vi "Main Engine Response LV2GBL.vi"(6 "Options":T1, 8 "error in":errorcluster) -> (0 "error out":errorcluster, 2 "Response":i32, 3 "Update":i32)   [LabVIEW 2021]
uses:
  Controls/Main Engine Engine No.Options.ctl
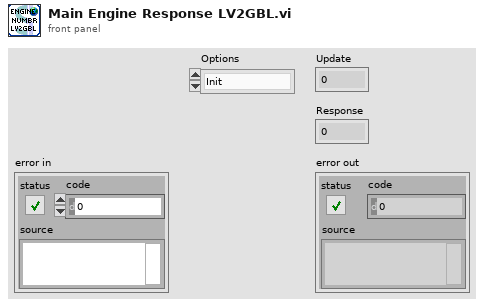
[diagram p1: front panel]
types:
  T1 = typedef "Main Engine Engine No.Options.ctl" = enum16{"Init", "Update", "Response", "Get"}
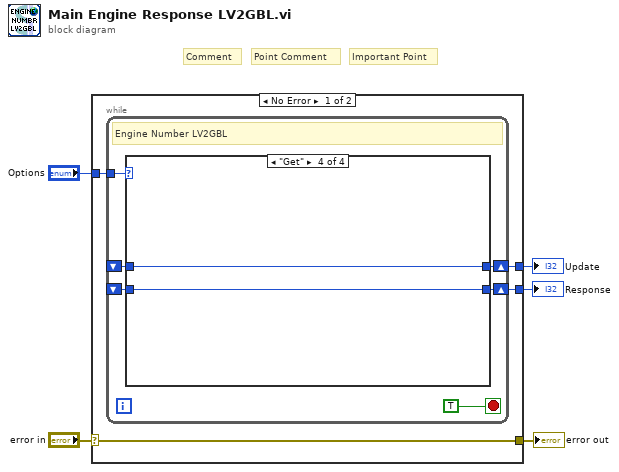
[diagram p0: block diagram]
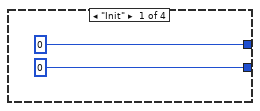
[diagram p2: hidden frame]
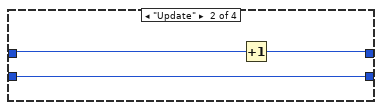
[diagram p3: hidden frame]
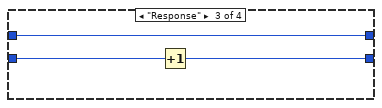
[diagram p4: hidden frame]
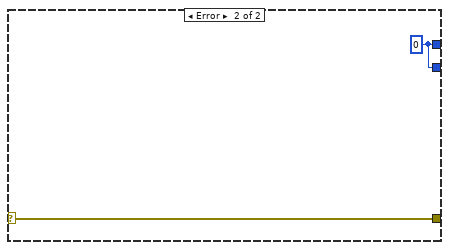
[diagram p5: hidden frame]
diagram:
  # "Important Point"
  # "Point Comment"
  # "Comment"
  n1 = case shown="No Error" "error in" {
    selector: "error in" -> [w8 w27]
    tunnel: "Options" -> [w9 _]
    tunnel: [w8 w27] -> w3
    tunnel: [w7 w26] -> w2
    tunnel: [w6 w26] -> w1
    frame No Error {
      n2 = while {
        tunnel: w9 -> [w14]
        shift-right: [w12] -> w6
        shift-left: _ -> [w10]
        shift-right: [w13] -> w7
        shift-left: _ -> [w11]
        stop <- TRUE stop-if-true
        # "Engine Number LV2GBL"
        n3 = case "Options?" shown="\"Get\"" w14 {
          tunnel: [0 w20 w21 w25] -> w13
          tunnel: [0 w18 w22 w24] -> w12
          tunnel: w11 -> [_ w19 w21 w25]
          tunnel: w10 -> [_ w18 w23 w24]
          frame "Init" {
          }
          frame "Update" {
            n4 = Increment(x=w19) -> (x+1=w20:i32)
          }
          frame "Response" {
            n5 = Increment(x=w23) -> (x+1=w22:i32)
          }
          frame "Get" {
          }
        }
      }
    }
    frame Error {
      w26 = 0
    }
  }
  "error out" <- w3
  "Update" <- w2
  "Response" <- w1
